vi "colored cells2.vi"() -> ()   [LabVIEW 2024]
uses:
  Grid/SourceGrid.lvclass
  Cells/Cell/Cell.lvclass
  System.Drawing.Color.ctl
  EDS-File-Viewer/source/Cell View Alternating Back Color/Cell View Alternating Back Color.lvclass
  SourceGrid.lvlib
  D:/git/Sourcegrid-LabVIEW/dll/SourceGrid.dll
  dll/SourceGrid.dll
panel:
  in  "Grid Container":refnum<k24>(container)
  in  "stop":bool
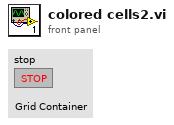
[diagram p1: front panel]
types:
  T1 = typedef "SourceGrid.lvlib/System.Drawing.Color.ctl" = enum16{"AliceBlue", "AntiqueWhite", "Aqua", "Aquamarine", "Azure", "Beige", "Bisque", "Black", "BlanchedAlmond", "Blue", "BlueViolet", "Brown", "BurlyWood", "CadetBlue", "Chartreuse", "Chocolate", "Coral", "CornflowerBlue", "Cornsilk", "Crimson", "Cyan", "DarkBlue", "DarkCyan", "DarkGoldenrod", "DarkGray", "DarkGreen", "DarkKhaki", "DarkMagenta", "DarkOliveGreen", "DarkOrange", "DarkOrchid", "DarkRed", "DarkSalmon", "DarkSeaGreen", "DarkSlateBlue", "DarkSlateGray", "DarkTurquoise", "DarkViolet", "DeepPink", "DeepSkyBlue", "DimGray", "DodgerBlue", "Firebrick", "FloralWhite", "ForestGreen", "Fuchsia", "Gainsboro", "GhostWhite", "Gold", "Goldenrod", "Gray", "Green", "GreenYellow", "Honeydew", "HotPink", "IndianRed", "Indigo", "Ivory", "Khaki", "Lavender", "LavenderBlush", "LawnGreen", "LemonChiffon", "LightBlue", "LightCoral", "LightCyan", "LightGoldenrodYellow", "LightGray", "LightGreen", "LightPink", "LightSalmon", "LightSeaGreen", "LightSkyBlue", "LightSlateGray", "LightSteelBlue", "LightYellow", "Lime", "LimeGreen", "Linen", "Magenta", "Maroon", "MediumAquamarine", "MediumBlue", "MediumOrchid", "MediumPurple", "MediumSeaGreen", "MediumSlateBlue", "MediumSpringGreen", "MediumTurquoise", "MediumVioletRed", "MidnightBlue", "MintCream", "MistyRose", "Moccasin", "NavajoWhite", "Navy", "OldLace", "Olive", "OliveDrab", "Orange", "OrangeRed", "Orchid", "PaleGoldenrod", "PaleGreen", "PaleTurquoise", "PaleVioletRed", "PapayaWhip", "PeachPuff", "Peru", "Pink", "Plum", "PowderBlue", "Purple", "Red", "RosyBrown", "RoyalBlue", "SaddleBrown", "Salmon", "SandyBrown", "SeaGreen", "SeaShell", "Sienna", "Silver", "SkyBlue", "SlateBlue", "SlateGray", "Snow", "SpringGreen", "SteelBlue", "Tan", "Teal", "Thistle", "Tomato", "Transparent", "Turquoise", "Violet", "Wheat", "White", "WhiteSmoke", "Yellow"}
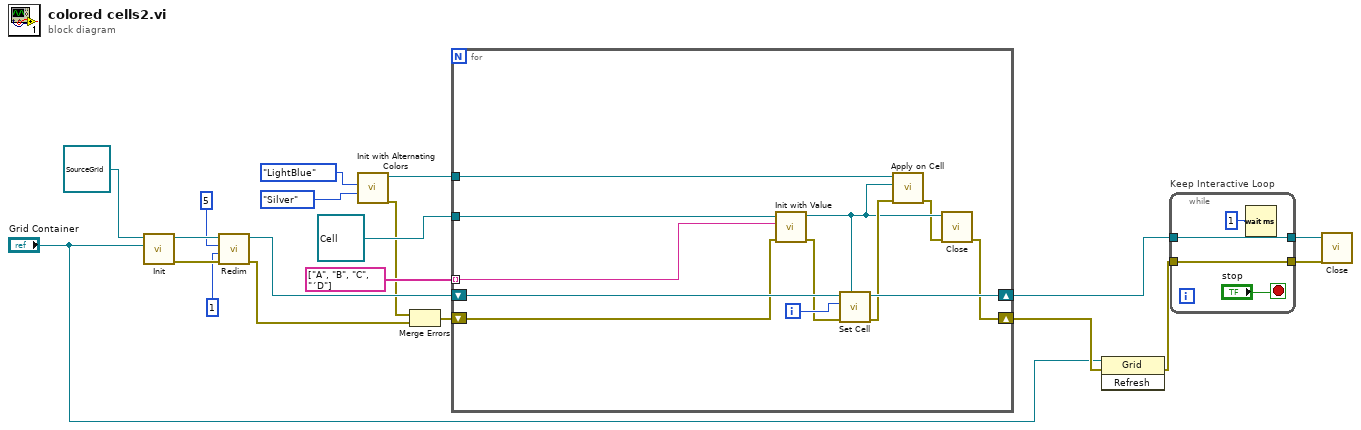
[diagram p0: block diagram]
diagram:
  n1 = call-dynamic "Init.vi"("Sourcegrid Container"="Grid Container", "Grid in"=refnum<class "SourceGrid.lvclass"> refnum) -> ("error out"=w17:errorcluster, "Grid out"=w15:refnum<class "SourceGrid.lvclass">)  [unwired: 8 in]
  n2 = call "Redim.vi"("error in"=w17, "Columns"=1, "Rows"=5, "Sourcegrid in"=w15) -> ("error out"=w12:errorcluster, "Sourcegrid out"=w11:refnum<class "SourceGrid.lvclass">)  [unwired: 6 in]
  n3 = call "Init with Alternating Colors.vi"("Color Not Equal"=System.Drawing.Color."Silver" ("Color"), "Color Equal"=System.Drawing.Color."LightBlue" ("Color")) -> ("error out"=w1:errorcluster, "Cell View Alternating Back Color out"=w3:refnum<class "Cell View Alternating Back Color.lvclass">)  [unwired: 8 in]
  n4 = Merge Errors(w1, w12) -> (w2:errorcluster)
  n5 = for {
    shift-right: [w29] -> w16
    shift-left: w11 -> [w32]
    shift-right: [w26] -> w10
    shift-left: w2 -> [w28]
    tunnel: w3 -> [w24]
    tunnel: refnum<class "Cell.lvclass"> refnum ("Cell in") -> [w25]
    tunnel: string[] ["A", "B", "C", "´D"] -> [w31] mode=indexing
    i -> [w30]
    n6 = call-dynamic "Init with Value.vi"("error in"=w28, "Value"=w31, "Cell in"=w25) -> ("error out"=w27:errorcluster, "Cell out"=w22:refnum<class "Cell.lvclass">)  [unwired: 7 in]
    n7 = call "Set Cell.vi"("Cell"=w22, "error in"=w27, "Row"=w30, "Sourcegrid in"=w32) -> ("error out"=w23:errorcluster, "Sourcegrid out"=w29:refnum<class "SourceGrid.lvclass">)  [unwired: 6 in]
    n8 = call-dynamic "Apply on Cell.vi"("error in"=w23, "Cell"=w22, "Cell View Alternating Back Color in"=w24) -> ("error out"=w21:errorcluster)  [unwired: 7 in, 1 out]
    n9 = call-dynamic "Close.vi"("error in"=w21, "Cell in"=w22) -> ("error out"=w26:errorcluster)  [unwired: 8 in, 1 out]
  }
  n10 = invoke class="Grid" method="Refresh"(reference="Grid Container", error in=w10) -> (error out=w9:errorcluster)  [unwired: 1 in, 2 out]
  n11 = while "Keep Interactive Loop" {
    tunnel: w16 -> [w36]
    tunnel: [w36] -> w20
    tunnel: w9 -> [w35]
    tunnel: [w35] -> w19
    stop <- "stop" stop-if-true
    n12 = Wait (ms)(milliseconds to wait=u32 1) -> ()  [unwired: 1 out]
  }
  n13 = call-dynamic "Close.vi"("error in"=w19, "Sourcegrid in"=w20) -> ()  [unwired: 8 in, 2 out]
